vi "Interfaz v0.vi"() -> ()   [LabVIEW 2011]
panel:
  in  "V Max Norte":dbl
  in  "V Min Norte":dbl
  in  "V Max Sur":dbl
  in  "V Min Sur":dbl
  in  "Rango de Control Sur (± T)":dbl
  in  "Rango de Control Norte (± T)":dbl
  out "Temperatura Sur":sgl(graph)
  out "V Norte":string
  in  "stop 2":bool
  out "Temperatura Norte":sgl(graph)
  out "V Sur":string
  in  "D":dbl=4.0
  in  "I":dbl=2.0
  in  "P":dbl=4.0
  in  "?":bool
  in  "?":bool
  in  "Fuente Sur":bool
  in  "Fuente Norte":bool
  out "Estado de la máquina":string
  in  "Fuente Sur":refnum<visa-resource-name>="COM1"
  out "Temperatura Norte":dbl
  out "Temperatura Sur":dbl
  in  "Temperatura Norte":dbl
  in  "Pico":refnum<visa-resource-name>="COM1"
  in  "Fuente Norte":refnum<visa-resource-name>="COM1"
  out "Norte":dbl(slide) scale=0.0..200.0
  out "Tiempo de ejecución":dbl
  in  "stop":bool
  out "Sur":dbl(slide) scale=0.0..100.0
  in  "Temperatura Sur":dbl
  # "Paso Previo:\n\nAntes de comenzar asignar un puerto a cada aparato:"
  # "VARIABLES"
  # "CONFIGURACIÓN\n\n\n\n\n\n\n\n\n\n\n\n\n\n\n\n\nPID Temperatura\n\n\n\n\n\n\nPID Deposición"
  # "Instrucciones:\n\nSeleccionar cada módulo que se quiere incluir en la experiencia.\n\nMódulo \"Fuente Sur\" -> Activa el control de la fuente Sur.\n\nMódulo \"Fuente Norte\" -> Activa el control de la fuente Norte.\n\nMódulo \"Balanza de Cuarzo\" -> Activa el control de la balanza."
  # "Módulo Fuente Sur:\n\nSeleccione la temperatura inicial \ndeseada en la placa Sur."
  # "Módulo Fuente Norte:\n\nSeleccione la temperatura inicial \ndeseada en la placa Sur."
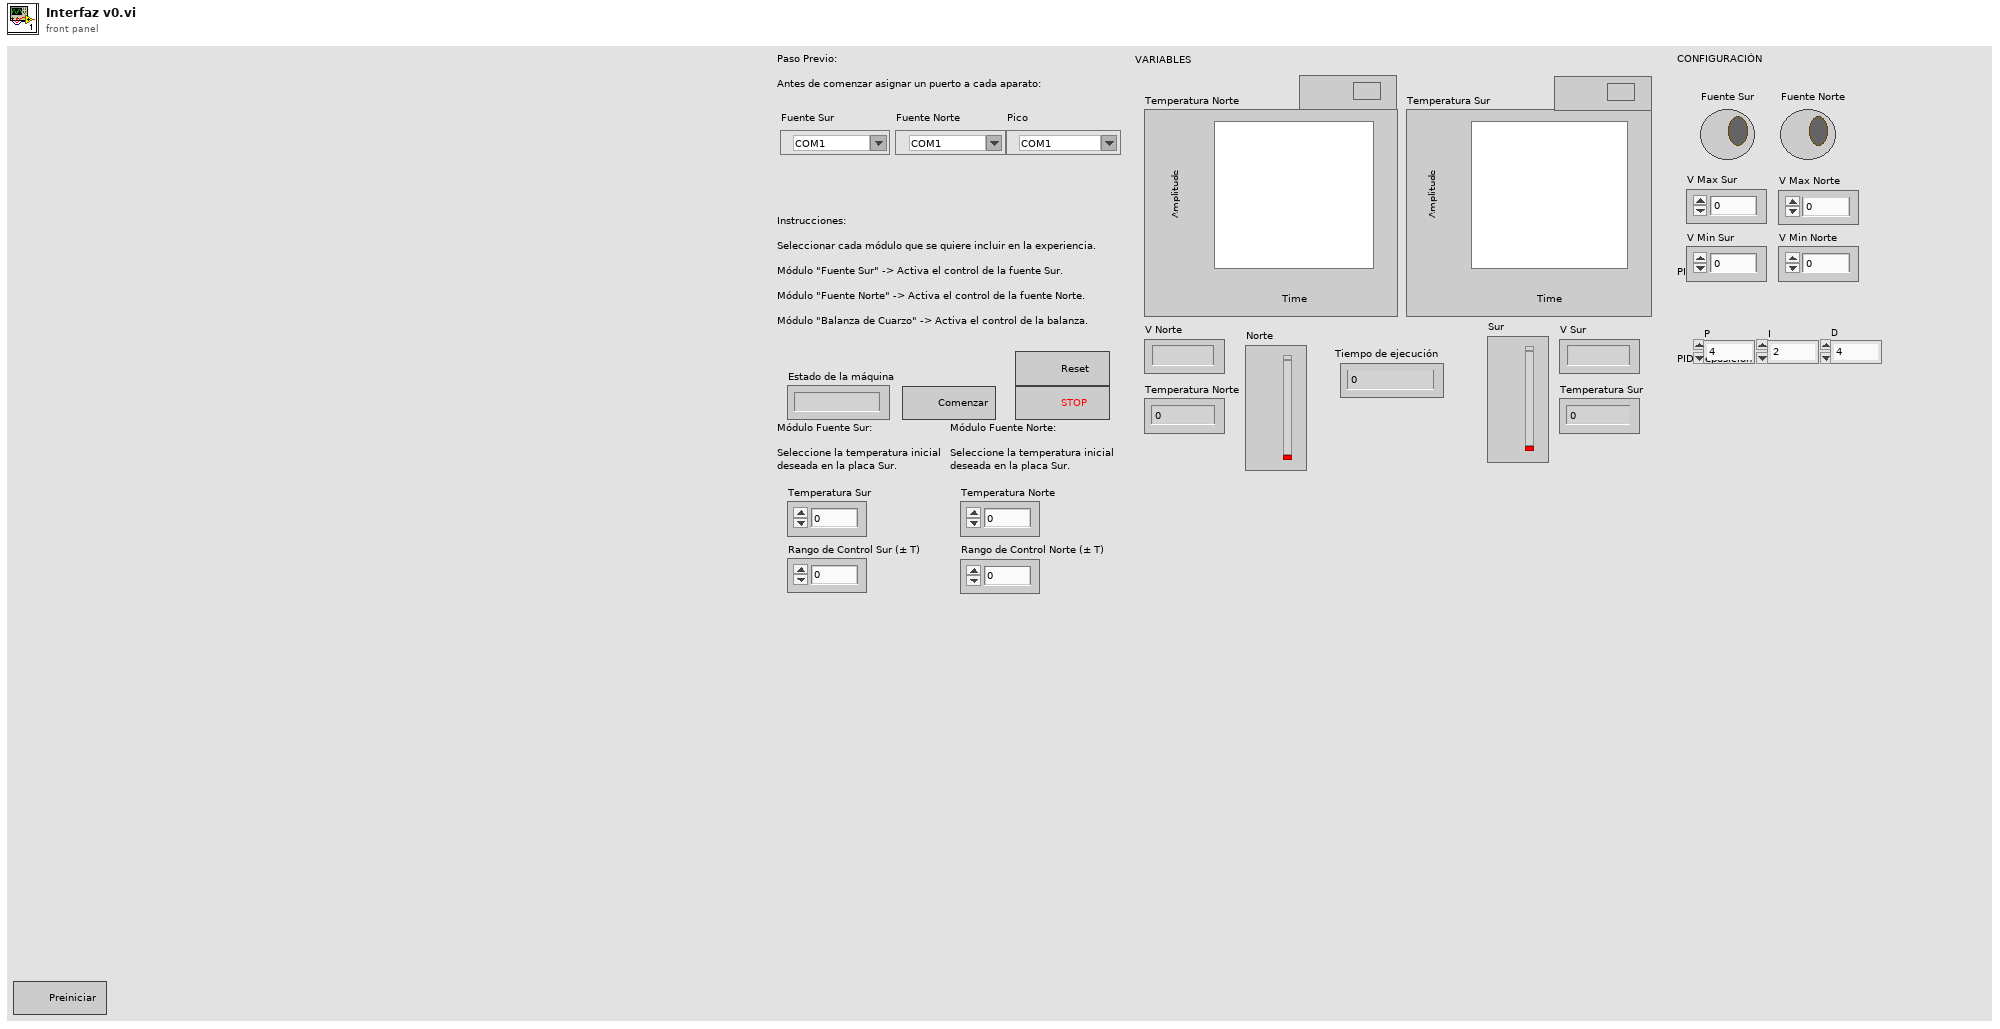
[diagram p1: front panel]
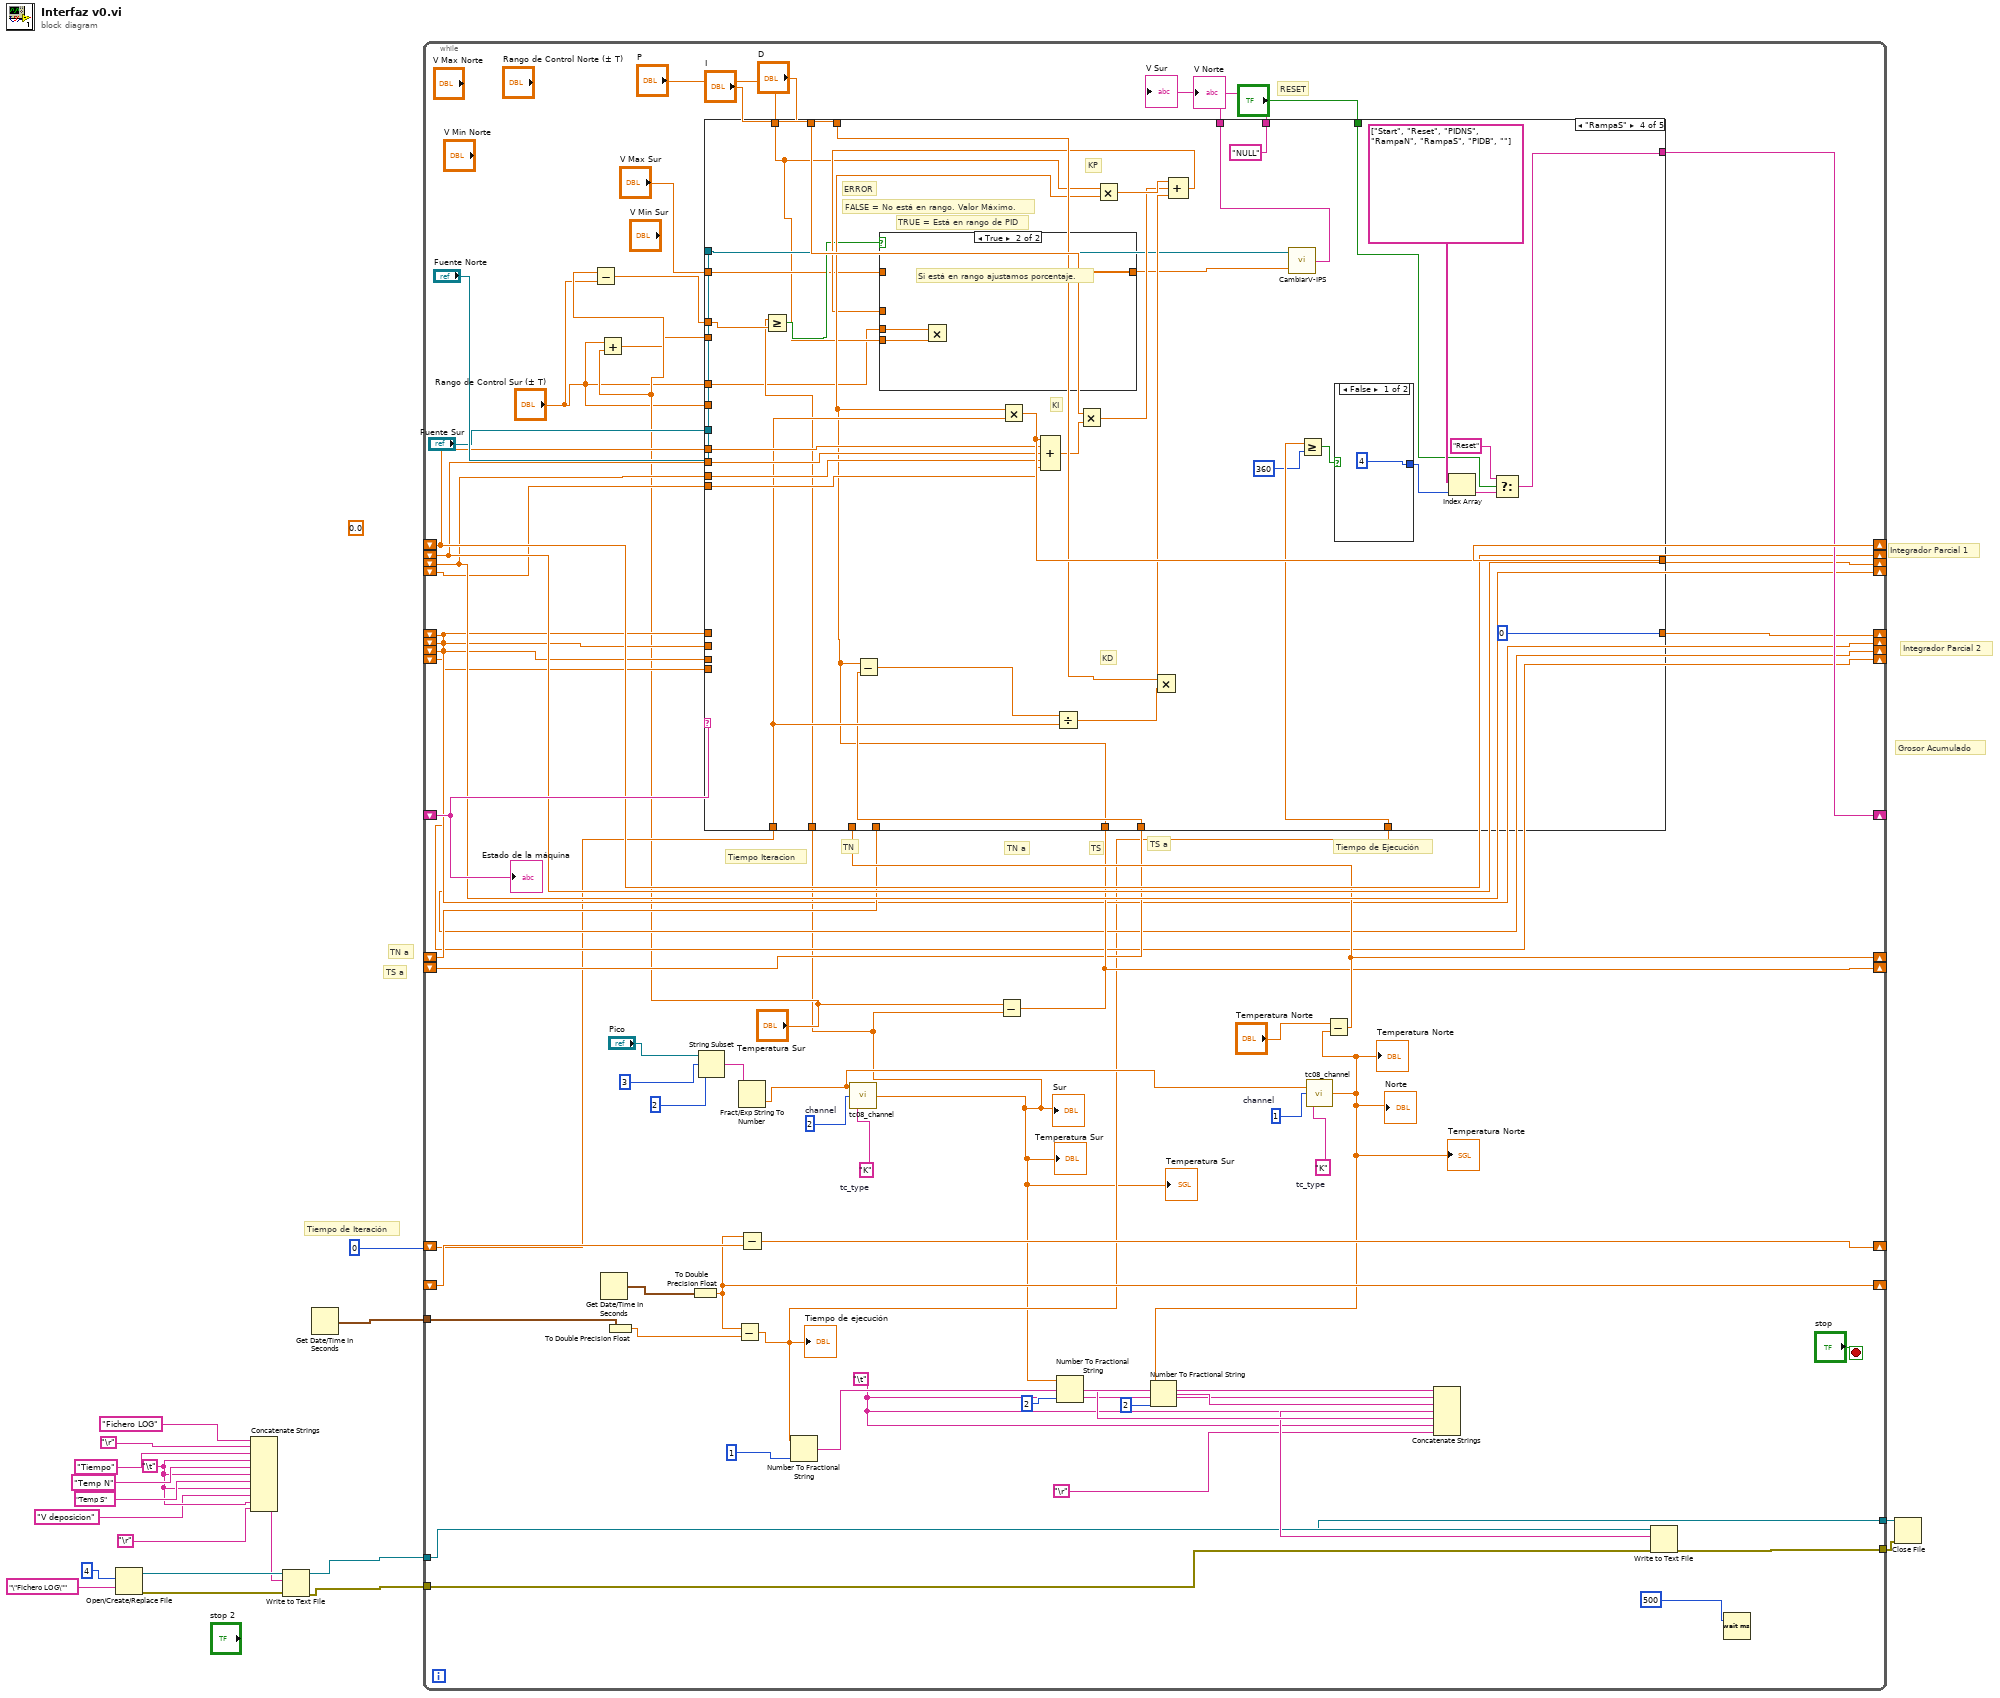
[diagram p0: block diagram]
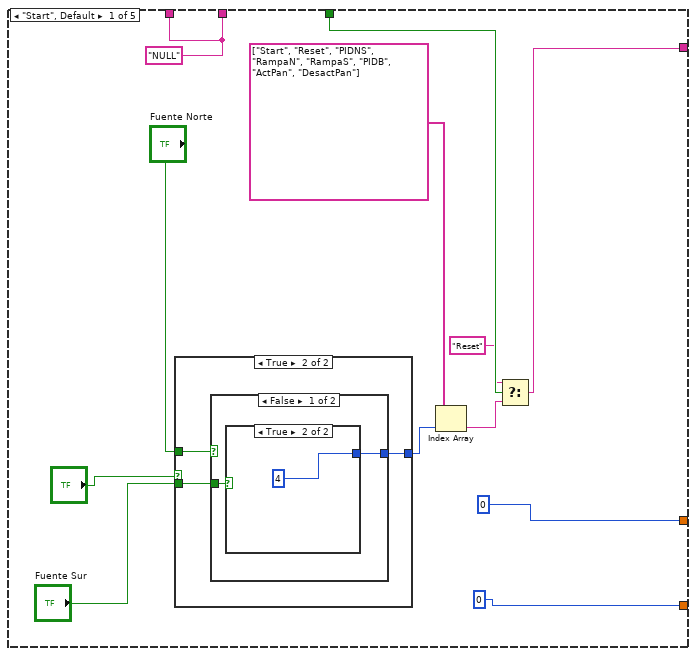
[diagram p2: hidden frame]
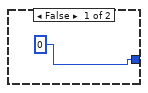
[diagram p3: hidden frame]
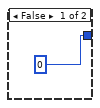
[diagram p4: hidden frame]
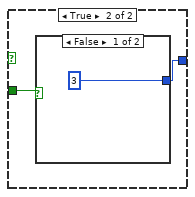
[diagram p5: hidden frame]
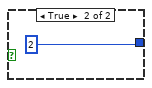
[diagram p6: hidden frame]
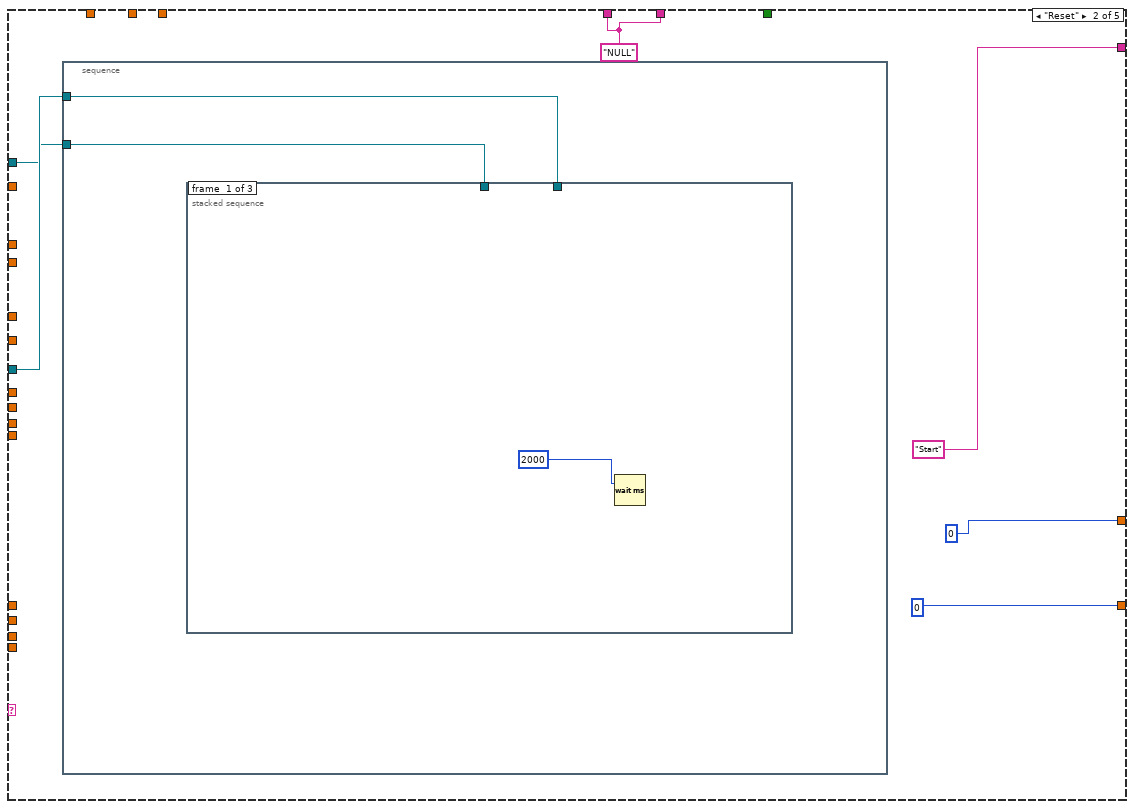
[diagram p7: hidden frame]
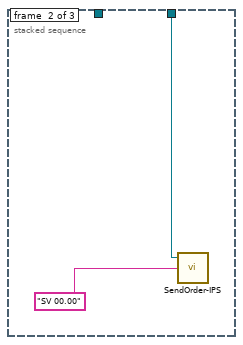
[diagram p8: hidden frame]
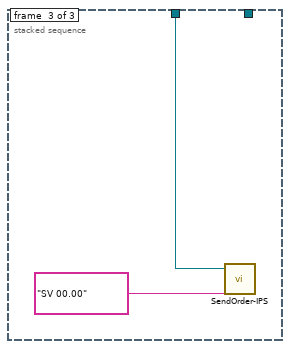
[diagram p9: hidden frame]
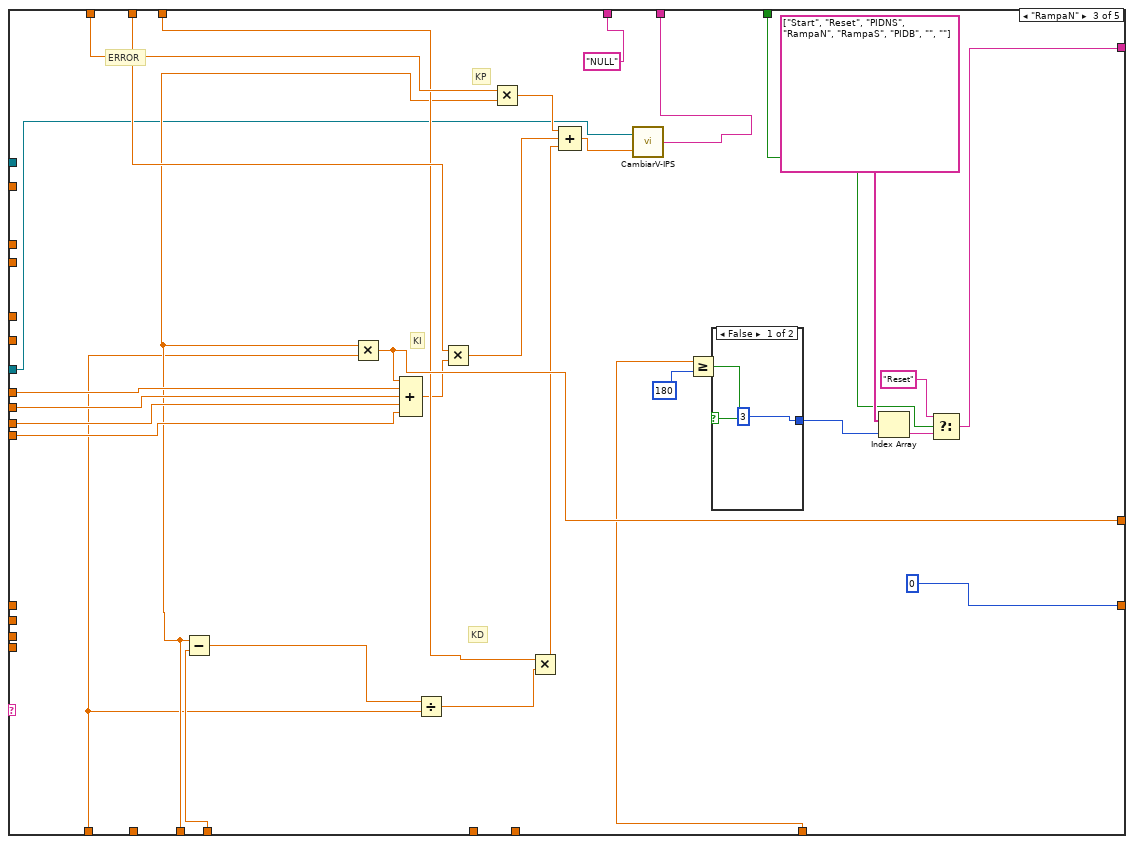
[diagram p10: hidden frame]
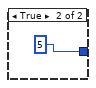
[diagram p11: hidden frame]
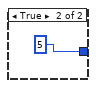
[diagram p13: hidden frame]
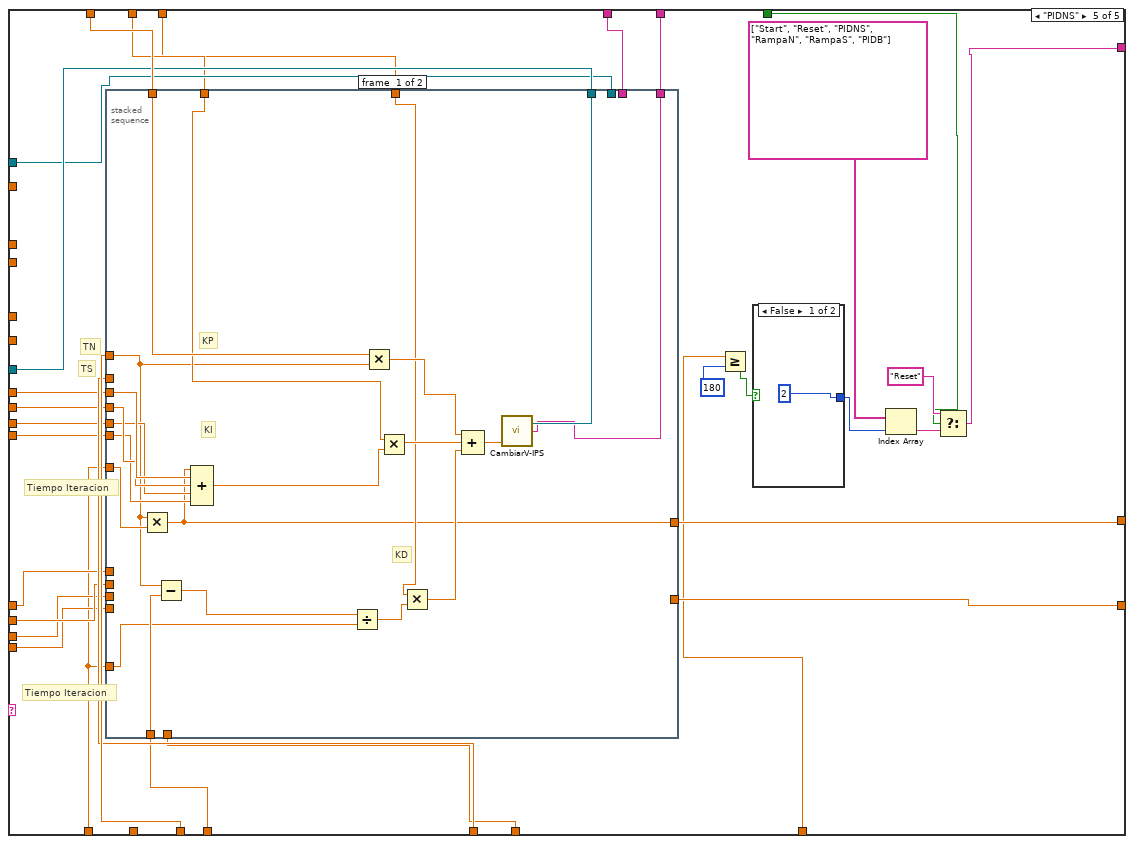
[diagram p14: hidden frame]
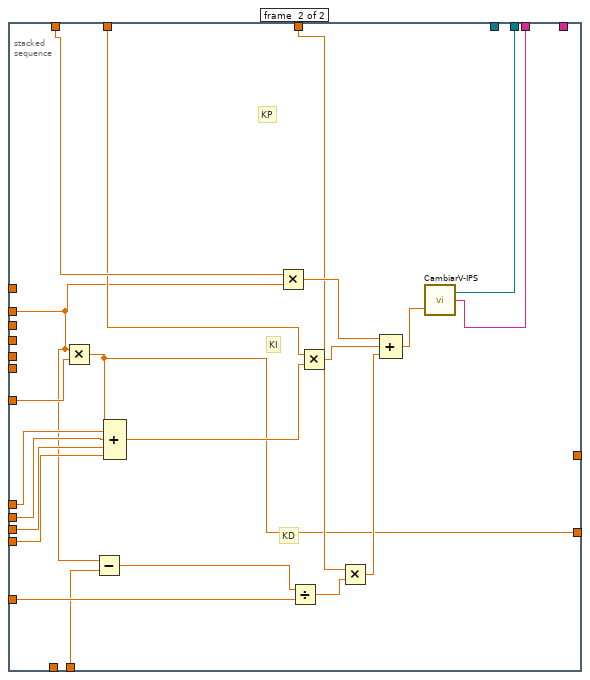
[diagram p15: hidden frame]
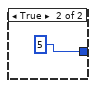
[diagram p16: hidden frame]
diagram:
  (unwired) 0.0
  w2 = "\t"
  # "Grosor Acumulado"
  # "Integrador Parcial 2"
  # "TS a"
  # "TN a"
  # "Integrador Parcial 1"
  # "Tiempo de Iteración"
  n1 = Open/Create/Replace File(prompt="\"Fichero LOG\"", operation (0:open)=4) -> (refnum out=w14:refnum<file>, error out=w13:errorcluster)  [unwired: 4 in, 1 out]
  n2 = Concatenate Strings("Fichero LOG", "\r", "Tiempo", w2, "Temp N", w2, "Temp S", w2, "V deposicion", w2, "\r") -> (w12:string)
  n3 = Write to Text File(file (use dialog)=w14, text=w12, error in=w13) -> (refnum out=w5:refnum<file>, error out=w4:errorcluster)  [unwired: 1 in, 1 out]
  n4 = Get Date/Time In Seconds() -> (seconds since 1Jan1904=w19:timestamp)
  n5 = while {
    shift-right: [w62] -> _
    shift-left: _ -> [w70]
    tunnel: w19 -> [w79]
    shift-right: [w76] -> _
    shift-left: _ -> [w77]
    shift-right: [w75] -> _
    shift-left: 0 -> [w27]
    shift-right: [w63] -> _
    shift-left: _ -> [w61]
    shift-right: [w61] -> _
    shift-left: _ -> [w60]
    shift-right: [w60] -> _
    shift-left: _ -> [w59]
    shift-right: [w59] -> _
    shift-left: _ -> [w58]
    shift-right: [w55] -> _
    shift-left: _ -> [w53]
    shift-right: [w54] -> _
    shift-left: _ -> [w52]
    tunnel: w5 -> [w43]
    tunnel: w4 -> [w42]
    tunnel: [w41] -> w17
    tunnel: [w40] -> w16
    shift-right: [w36] -> _
    shift-left: _ -> [w35]
    shift-right: [w35] -> _
    shift-left: _ -> [w33]
    shift-right: [w33] -> _
    shift-left: _ -> [w34]
    shift-right: [w34] -> _
    shift-left: _ -> [w32]
    stop <- "stop" stop-if-true
    w28 = "\t"
    w73 = "K"  # tc_type
    w74 = u16 1  # channel
    w81 = "K"  # tc_type
    w82 = u16 2  # channel
    # "RESET"
    # "Tiempo de Ejecución"
    # "TS a"
    # "TN a"
    # "TS"
    # "Tiempo Iteracion"
    # "TN"
    n6 = Subtract(x="Temperatura Sur", y="Rango de Control Sur (± T)") -> (x-y=w24:dbl)
    n7 = Add(x="Rango de Control Sur (± T)", y="Temperatura Sur") -> (x+y=w23:dbl)
    n8 = Get Date/Time In Seconds() -> (seconds since 1Jan1904=w80:timestamp)
    n9 = To Double Precision Float(number=w79) -> (double precision float=w78:dbl)
    n10 = To Double Precision Float(number=w80) -> (double precision float=w76:dbl)
    n11 = String Subset(string="Pico", offset (0)=3, length (rest)=2) -> (substring=w66:string)
    n12 = Subtract(x=w76, y=w78) -> (x-y=w31:dbl)
    "Tiempo de ejecución" <- w31
    n13 = Fract/Exp String To Number(string=w66) -> (number=w37:dbl)  [unwired: 3 in, 1 out]
    n14 = Subtract(x=w76, y=w77) -> (x-y=w75:dbl)
    n15 = Number To Fractional String(number=w31, precision (6)=1) -> (F-format string=w51:string)  [unwired: 2 in]
    n16 = call "tc08_channel.vi"("tc_type"=w81, "channel"=w82, "port"=w37) -> ("Temperature"=w22:sgl)
    "Sur" <- w22
    "Temperatura Sur" <- w22
    "Temperatura Sur" <- w22
    n17 = Subtract(x="Temperatura Sur", y=w22) -> (x-y=w54:dbl)
    n18 = Number To Fractional String(number=w22, precision (6)=2) -> (F-format string=w49:string)  [unwired: 2 in]
    n19 = call "tc08_channel.vi"("tc_type"=w73, "channel"=w74, "port"=w37) -> ("Temperature"=w46:sgl)
    "Norte" <- w46
    "Temperatura Norte" <- w46
    "Temperatura Norte" <- w46
    n20 = Number To Fractional String(number=w46, precision (6)=2) -> (F-format string=w47:string)  [unwired: 2 in]
    n21 = Subtract(x="Temperatura Norte", y=w46) -> (x-y=w55:dbl)
    n22 = case shown="\"RampaS\"" w70 {
      tunnel: [w90 "Start" w129 w170 w203] -> w62
      tunnel: "Fuente Norte" -> [_ w112 w134 _ w221]
      tunnel: "Fuente Sur" -> [_ w111 _ w175 w220]
      tunnel: "?" -> [w89 _ w127 w168 w201]
      tunnel: w55 -> [_ _ w138 _ w223]
      tunnel: w54 -> [_ _ _ w176 w222]
      tunnel: "P" -> [_ _ w151 w155 w224]
      tunnel: "I" -> [_ _ w149 w189 w210]
      tunnel: w27 -> [_ _ w136 w178 w211]
      tunnel: [0 0 w148 w188 w206] -> w63
      tunnel: w61 -> [_ _ w147 w187 w219]
      tunnel: w60 -> [_ _ w146 w186 w218]
      tunnel: w59 -> [_ _ w145 w185 w217]
      tunnel: w58 -> [_ _ w144 w184 w216]
      tunnel: "D" -> [_ _ w140 w180 w209]
      tunnel: w53 -> [_ _ w137 _ w208]
      tunnel: w52 -> [_ _ _ w177 w207]
      tunnel: [0 0 0 0 w205] -> w36
      tunnel: w35 -> [_ _ _ _ w215]
      tunnel: w34 -> [_ _ _ _ w213]
      tunnel: w33 -> [_ _ _ _ w214]
      tunnel: w32 -> [_ _ _ _ w212]
      tunnel: w31 -> [_ _ w123 w165 w198]
      tunnel: [w84 w108 w122 "NULL" w196] -> w30
      tunnel: [w84 w108 "NULL" w164 w197] -> w29
      tunnel: "Rango de Control Sur (± T)" -> [_ _ _ _ _]
      tunnel: w24 -> [_ _ _ w161 _]
      tunnel: w23 -> [_ _ _ _ _]
      tunnel: w22 -> [_ _ _ w160 _]
      tunnel: "V Max Sur" -> [_ _ _ w156 _]
      tunnel: "Rango de Control Sur (± T)" -> [_ _ _ w154 _]
      frame "Start", Default {
        w84 = "NULL"
        n23 = case shown="True" "?" {
          tunnel: [0 w99] -> w94
          tunnel: "Fuente Norte" -> [_ w98]
          tunnel: "Fuente Sur" -> [_ w97]
          frame False {
          }
          frame True {
            n24 = case shown="False" w98 {
              tunnel: [w100 w104] -> w99
              tunnel: w97 -> [w101 w105]
              frame False {
                n25 = case shown="True" w101 {
                  tunnel: [0 4] -> w100
                  frame False {
                  }
                  frame True {
                  }
                }
              }
              frame True {
                n26 = case shown="False" w105 {
                  tunnel: [3 2] -> w104
                  frame False {
                  }
                  frame True {
                  }
                }
              }
            }
          }
        }
        n27 = Index Array(array=string[] ["Start", "Reset", "PIDNS", "RampaN", "RampaS", "PIDB", "ActPan", "DesactPan"], index=w94) -> (element=w88:string)
        n28 = Select(t="Reset", s=w89, f=w88) -> (s? t:f=w90:string)
      }
      frame "Reset" {
        w108 = "NULL"
        n29 = stacked-sequence {
          tunnel: w112 -> [w115]
          tunnel: w111 -> [w114]
          frame #0 {
            n30 = stacked-sequence {
              tunnel: w115 -> [_ w118 _]
              tunnel: w114 -> [_ _ w120]
              frame #0 {
                n31 = Wait (ms)(milliseconds to wait=2000) -> ()  [unwired: 1 out]
              }
              frame #1 {
                n32 = call "SendOrder-IPS.vi"("string to write"="SV 00.00", "VISA resource name"=w118) -> ()  [unwired: 1 in, 1 out]
              }
              frame #2 {
                n33 = call "SendOrder-IPS.vi"("string to write"="SV 00.00", "VISA resource name"=w120) -> ()  [unwired: 1 in, 1 out]
              }
            }
          }
        }
      }
      frame "RampaN" {
        # "KD"
        # "ERROR"
        # "KI"
        # "KP"
        n34 = Subtract(x=w138, y=w137) -> (x-y=w141:dbl)
        n35 = Multiply(x=w138, y=w136) -> (x*y=w148:dbl)
        n36 = Compound Arithmetic op=ADD(w148, w147, w146, w145, w144) -> (w124:dbl)
        n37 = Divide(x=w141, y=w136) -> (x/y=w142:dbl)
        n38 = Multiply(x=w149, y=w124) -> (x*y=w143:dbl)
        n39 = Multiply(x=w151, y=w138) -> (x*y=w150:dbl)
        n40 = Multiply(x=w140, y=w142) -> (x*y=w139:dbl)
        n41 = Compound Arithmetic op=ADD(w150, w143, w139) -> (w135:dbl)
        n42 = call "CambiarV-IPS.vi"("Numeric"=w135, "VISA resource name"=w134) -> ("Voltios"=w122:string)
        n43 = Greater Or Equal?(x=w123, y=180) -> (x >= y?=w126:bool)
        n44 = case shown="False" w126 {
          tunnel: [3 5] -> w132
          frame False {
          }
          frame True {
          }
        }
        n45 = Index Array(array=string[] ["Start", "Reset", "PIDNS", "RampaN", "RampaS", "PIDB", "", ""], index=w132) -> (element=w130:string)
        n46 = Select(t="Reset", s=w127, f=w130) -> (s? t:f=w129:string)
      }
      frame "RampaS" {
        # "FALSE = No está en rango. Valor Máximo."
        # "TRUE = Está en rango de PID"
        # "ERROR"
        # "KD"
        # "KI"
        # "KP"
        n47 = Greater Or Equal?(x=w160, y=w161) -> (x >= y?=w157:bool)
        n48 = Subtract(x=w176, y=w177) -> (x-y=w181:dbl)
        n49 = Multiply(x=w176, y=w178) -> (x*y=w188:dbl)
        n50 = Compound Arithmetic op=ADD(w188, w187, w186, w185, w184) -> (w167:dbl)
        n51 = Divide(x=w181, y=w178) -> (x/y=w182:dbl)
        n52 = Multiply(x=w189, y=w167) -> (x*y=w183:dbl)
        n53 = Multiply(x=w155, y=w176) -> (x*y=w190:dbl)
        n54 = Multiply(x=w180, y=w182) -> (x*y=w179:dbl)
        n55 = Compound Arithmetic op=ADD(w190, w183, w179) -> (w159:dbl)
        n56 = case shown="True" w157 {
          tunnel: w159 -> [_ _]
          tunnel: [w191 _] -> w158
          tunnel: w156 -> [w191 _]
          tunnel: w155 -> [_ w193]
          tunnel: w154 -> [_ w192]
          frame False {
          }
          frame True {
            # "Si está en rango ajustamos porcentaje."
            n57 = Multiply(x=w192, y=w193) -> ()  [unwired: 1 out]
          }
        }
        n58 = call "CambiarV-IPS.vi"("Numeric"=w158, "VISA resource name"=w175) -> ("Voltios"=w164:string)
        n59 = Greater Or Equal?(x=w165, y=360) -> (x >= y?=w166:bool)
        n60 = case shown="False" w166 {
          tunnel: [4 5] -> w173
          frame False {
          }
          frame True {
          }
        }
        n61 = Index Array(array=string[] ["Start", "Reset", "PIDNS", "RampaN", "RampaS", "PIDB", ""], index=w173) -> (element=w171:string)
        n62 = Select(t="Reset", s=w168, f=w171) -> (s? t:f=w170:string)
      }
      frame "PIDNS" {
        # "Tiempo Iteracion"
        # "Tiempo Iteracion"
        # "TS"
        # "TN"
        n63 = stacked-sequence {
          tunnel: w224 -> [w246 w267]
          tunnel: w223 -> [w232 _]
          tunnel: w222 -> [_ w252]
          tunnel: w221 -> [w244 _]
          tunnel: w220 -> [_ w265]
          tunnel: w219 -> [w241 _]
          tunnel: w218 -> [w240 _]
          tunnel: w217 -> [w239 _]
          tunnel: w216 -> [w238 _]
          tunnel: w215 -> [_ w262]
          tunnel: w214 -> [_ w261]
          tunnel: w213 -> [_ w260]
          tunnel: w212 -> [_ w259]
          tunnel: w211 -> [w230 w254]
          tunnel: w211 -> [w237 w258]
          tunnel: w210 -> [w234 w257]
          tunnel: w209 -> [w233 w251]
          tunnel: w208 -> [w231 _]
          tunnel: w207 -> [_ w253]
          tunnel: [w228 _] -> w206
          tunnel: [_ w249] -> w205
          tunnel: [_ w248] -> w197
          tunnel: [w227 _] -> w196
          frame #0 {
            # "KD"
            # "KI"
            # "KP"
            n64 = Multiply(x=w232, y=w237) -> (x*y=w228:dbl)
            n65 = Subtract(x=w232, y=w231) -> (x-y=w235:dbl)
            n66 = Compound Arithmetic op=ADD(w228, w241, w240, w239, w238) -> (w243:dbl)
            n67 = Divide(x=w235, y=w230) -> (x/y=w236:dbl)
            n68 = Multiply(x=w246, y=w232) -> (x*y=w247:dbl)
            n69 = Multiply(x=w234, y=w243) -> (x*y=w242:dbl)
            n70 = Multiply(x=w233, y=w236) -> (x*y=w229:dbl)
            n71 = Compound Arithmetic op=ADD(w247, w242, w229) -> (w245:dbl)
            n72 = call "CambiarV-IPS.vi"("Numeric"=w245, "VISA resource name"=w244) -> ("Voltios"=w227:string)
          }
          frame #1 {
            # "KD"
            # "KI"
            # "KP"
            n73 = Multiply(x=w252, y=w258) -> (x*y=w249:dbl)
            n74 = Subtract(x=w252, y=w253) -> (x-y=w256:dbl)
            n75 = Compound Arithmetic op=ADD(w249, w262, w261, w260, w259) -> (w264:dbl)
            n76 = Multiply(x=w267, y=w252) -> (x*y=w268:dbl)
            n77 = Divide(x=w256, y=w254) -> (x/y=w255:dbl)
            n78 = Multiply(x=w257, y=w264) -> (x*y=w263:dbl)
            n79 = Multiply(x=w251, y=w255) -> (x*y=w250:dbl)
            n80 = Compound Arithmetic op=ADD(w268, w263, w250) -> (w266:dbl)
            n81 = call "CambiarV-IPS.vi"("Numeric"=w266, "VISA resource name"=w265) -> ("Voltios"=w248:string)
          }
        }
        n82 = Greater Or Equal?(x=w198, y=180) -> (x >= y?=w199:bool)
        n83 = case shown="False" w199 {
          tunnel: [2 5] -> w226
          frame False {
          }
          frame True {
          }
        }
        n84 = Index Array(array=string[] ["Start", "Reset", "PIDNS", "RampaN", "RampaS", "PIDB"], index=w226) -> (element=w202:string)
        n85 = Select(t="Reset", s=w201, f=w202) -> (s? t:f=w203:string)
      }
    }
    "V Norte" <- w30
    "V Sur" <- w29
    n86 = Concatenate Strings(w51, w28, w47, w28, w49, w28, "\r") -> (w44:string)
    n87 = Write to Text File(file (use dialog)=w43, text=w44, error in=w42) -> (refnum out=w41:refnum<file>, error out=w40:errorcluster)  [unwired: 1 in, 1 out]
    n88 = Wait (ms)(milliseconds to wait=500) -> ()  [unwired: 1 out]
    "Estado de la máquina" <- w70
  }
  n89 = Close File(refnum=w17, error in=w16) -> ()  [unwired: 2 out]
